vi "Car_TemplateMethod.vi"(8 "ErrorIn":errorcluster, 10 "CmdData":variant, 11 "Car:Car in":refnum<class>) -> (0 "ErrorOut":errorcluster, 2 "ReplyData":variant, 3 "Car:Car out":refnum<class>, 4 "Exit":bool)   [LabVIEW 2021, in "Car.lvlib" / "Car.lvclass"]
uses:
  Car.lvclass
  Car.lvclass/Car.ctl
  C:/Localdata/Projects/TriekselSoft/TriekselsoftApplicationFramework/Source/.Externals/Library_YAF/YAFTAF/YAFTAF.lvclass
  C:/Localdata/Projects/TriekselSoft/TriekselsoftApplicationFramework/Source/.Externals/Library_YAF/YActor/YActor.lvclass
  C:/Localdata/Projects/TriekselSoft/TriekselsoftApplicationFramework/Source/.Externals/Interface_UserInterface_IFrontPanel/IFrontPanel/IFrontPanel.lvclass
  C:/Localdata/Projects/TriekselSoft/TriekselsoftApplicationFramework/Source/.Externals/Interface_TAF_IInterface/IInterface/IInterface.lvclass
  C:/Localdata/Projects/TriekselSoft/TriekselsoftApplicationFramework/Source/.Externals/Interface_Object_ICreateDestroy/ICreateDestroy/ICreateDestroy.lvclass
  C:/Localdata/Projects/TriekselSoft/TriekselsoftApplicationFramework/Source/.Externals/Interface_Object_IPersistentData/IPersistentData/IPersistentData.lvclass
  C:/Localdata/Projects/TriekselSoft/TriekselsoftApplicationFramework/Source/.Externals/Interface_TAF_ITAFObject/ITAFObject/ITAFObject.lvclass
  C:/Localdata/Projects/TriekselSoft/TriekselsoftApplicationFramework/Documentation/Project Documentation/ExampleCode/Car/Car.lvclass
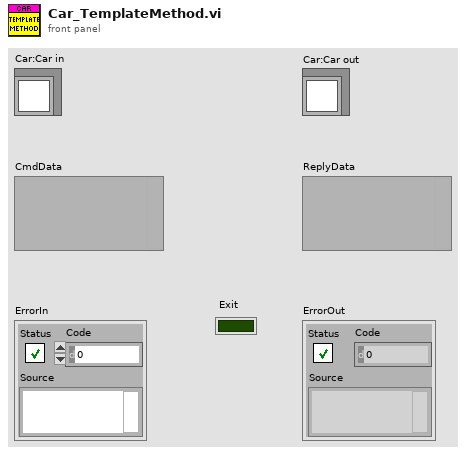
[diagram p1: front panel]
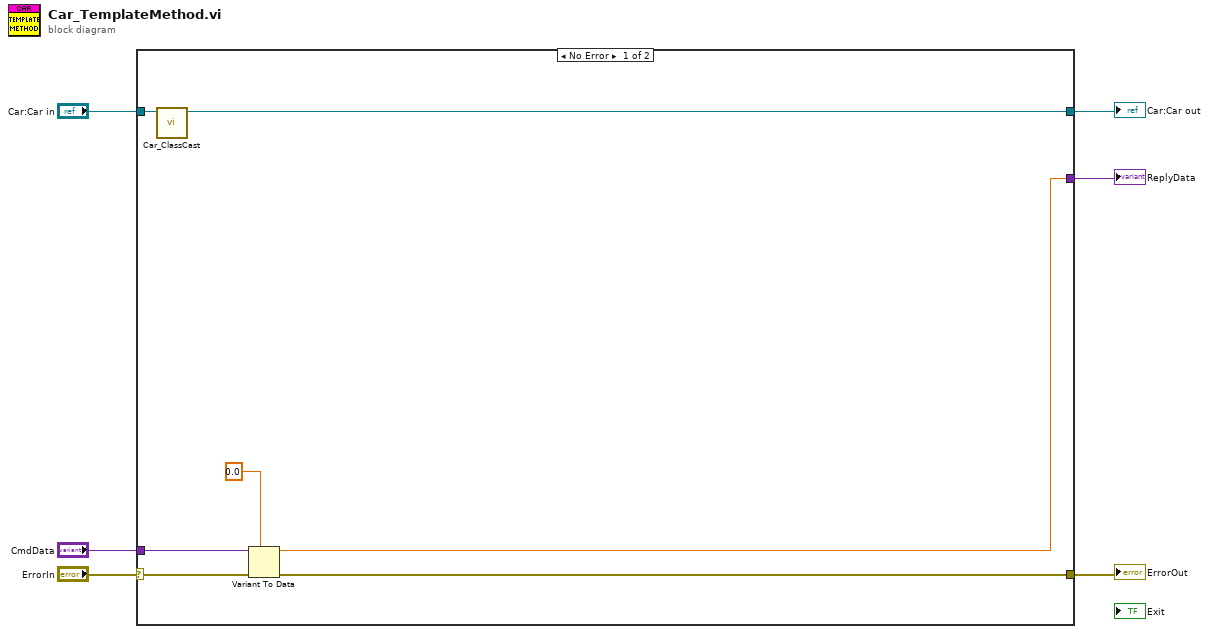
[diagram p0: block diagram]
diagram:
  n1 = case shown="No Error" "ErrorIn" {
    selector: "ErrorIn" -> [w13 w16]
    tunnel: [w12 w16] -> w5
    tunnel: [w7 w15] -> w3
    tunnel: "CmdData" -> [w10 w15]
    tunnel: "Car:Car in" -> [w11 w14]
    tunnel: [w9 w14] -> w1
    frame No Error {
      n2 = call "Car_ClassCast.vi"("Car:Car in"=w11) -> ("Car:Car out"=w9:refnum<class "Car.lvclass">)  [unwired: 10 in]
      n3 = Variant To Data(error in=w13, type=0.0 ("DummyIn"), Variant=w10) -> (data=w7:dbl, error out=w12:errorcluster)
    }
    frame Error {
    }
  }
  "ErrorOut" <- w5
  "Car:Car out" <- w1
  "ReplyData" <- w3
